vi "mytimer3.vi"() -> ()   [LabVIEW 2018]
panel:
  in  "Auto Reset":bool
  in  "Reset":bool
  out "Time Elapsed":dbl
  out "target achieved":bool
  in  "target":dbl
  in  "?":bool
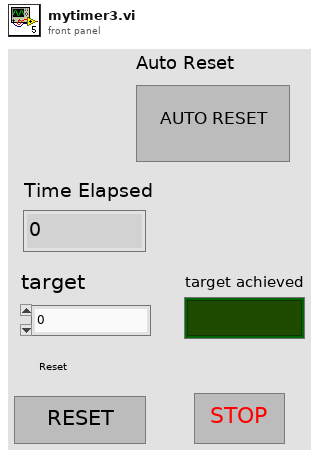
[diagram p1: front panel]
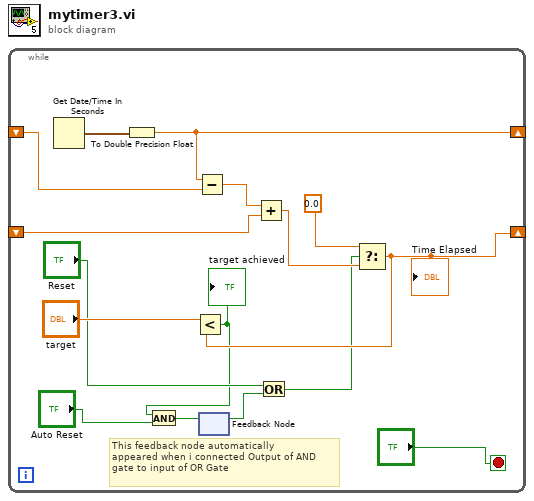
[diagram p0: block diagram]
diagram:
  n1 = while {
    shift-right: [w15] -> _
    shift-left: _ -> [w14]
    shift-right: [w9] -> _
    shift-left: _ -> [w11]
    stop <- "?" stop-if-true
    # "This feedback node automatically\nappeared when i connected Output of AND gate to input of OR Gate"
    n2 = Get Date/Time In Seconds() -> (seconds since 1Jan1904=w16:timestamp)
    n3 = To Double Precision Float(number=w16) -> (double precision float=w15:dbl)
    n4 = Subtract(x=w15, y=w14) -> (x-y=w13:dbl)
    n5 = feedback #1() -> (w1:bool)  [unwired: 1 in]
    n6 = Add(x=w13, y=w11) -> (x+y=w10:dbl)
    n7 = Or(x="Reset", y=w1) -> (x .or. y?=w5:bool)
    n8 = Select(t=0.0, s=w5, f=w10) -> (s? t:f=w9:dbl)
    "Time Elapsed" <- w9
    n9 = Less?(x="target", y=w9) -> (x < y?=w3:bool)
    "target achieved" <- w3
    n10 = And(x=w3, y="Auto Reset") -> (x .and. y?=w2:bool)
    n11 = feedback-in #1(w2) -> ()
  }
